vi "Write Num of boids.vi"(8 "error in (no error)":errorcluster, 10 "Num of boids":i32=50, 11 "Swiat in":refnum<class "Swiat.lvclass">) -> (0 "error out":errorcluster, 3 "Swiat out":refnum<class "Swiat.lvclass">)   [LabVIEW 2014, in "Swiat.lvclass"]
uses:
  Swiat.lvclass
  Swiat.lvclass/Swiat.ctl
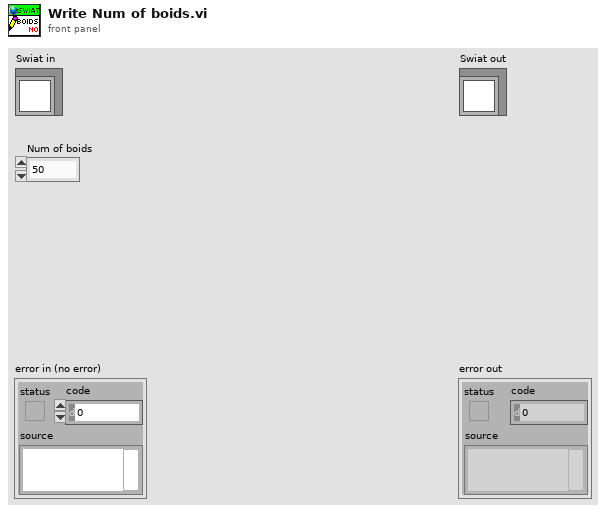
[diagram p1: front panel]
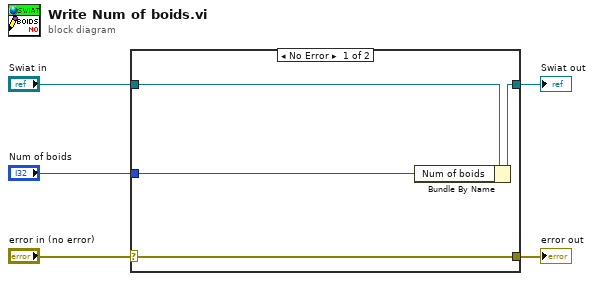
[diagram p0: block diagram]
diagram:
  n1 = case shown="No Error" "error in (no error)" {
    selector: "error in (no error)" -> [w9 w10]
    tunnel: [w9 w10] -> w4
    tunnel: [w7 w11] -> w2
    tunnel: "Swiat in" -> [w8 w11]
    tunnel: "Num of boids" -> [w6 _]
    frame No Error {
      n2 = Bundle By Name(cluster=w8, "Num of boids"=w6) -> (w7:refnum<class "Swiat.lvclass">)
    }
    frame Error {
    }
  }
  "error out" <- w4
  "Swiat out" <- w2
